vi "set optimum range.vi"(0 "denge degeri":dbl) -> (15 "ok":bool)   [LabVIEW 2014]
uses:
  Sub_VI/show_sensitivity.vi
panel:
  out "cycle":bool
  in  "GPIB In":refnum<visa-resource-name>="GPIB0::8::INSTR"
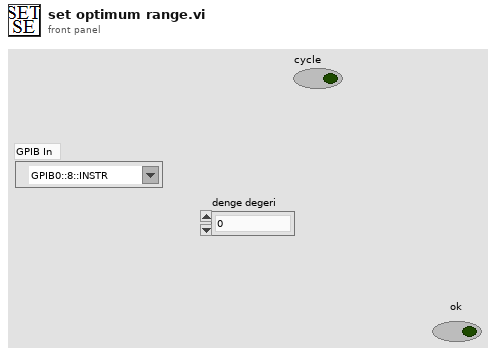
[diagram p1: front panel]
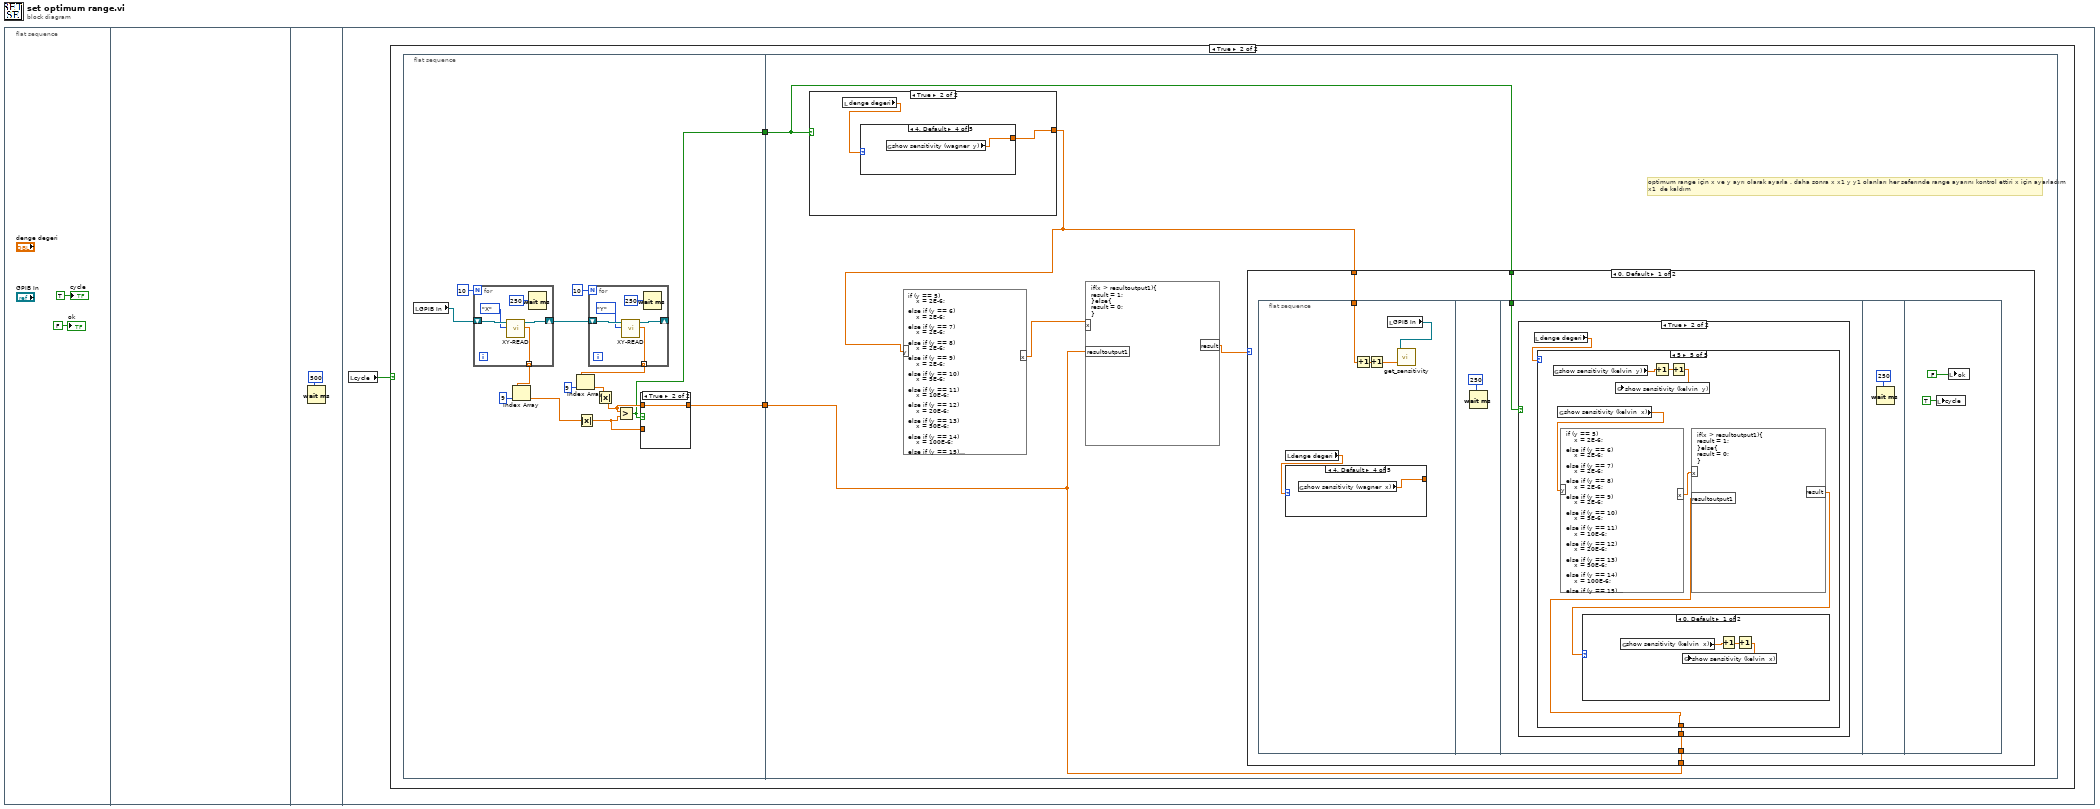
[diagram p0: block diagram]
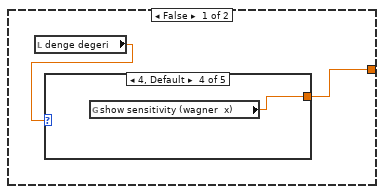
[diagram p4: hidden frame]
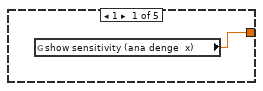
[diagram p5: hidden frame]
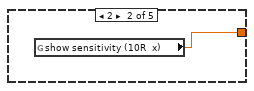
[diagram p6: hidden frame]
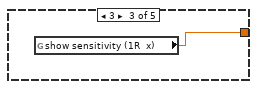
[diagram p7: hidden frame]
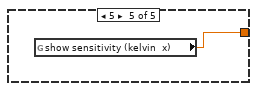
[diagram p8: hidden frame]
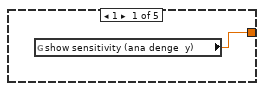
[diagram p9: hidden frame]
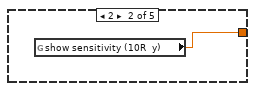
[diagram p10: hidden frame]
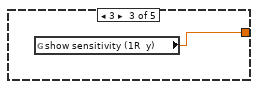
[diagram p11: hidden frame]
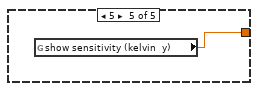
[diagram p12: hidden frame]
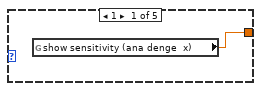
[diagram p13: hidden frame]
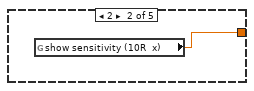
[diagram p14: hidden frame]
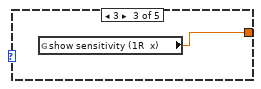
[diagram p15: hidden frame]
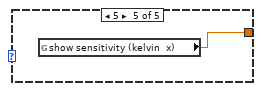
[diagram p16: hidden frame]
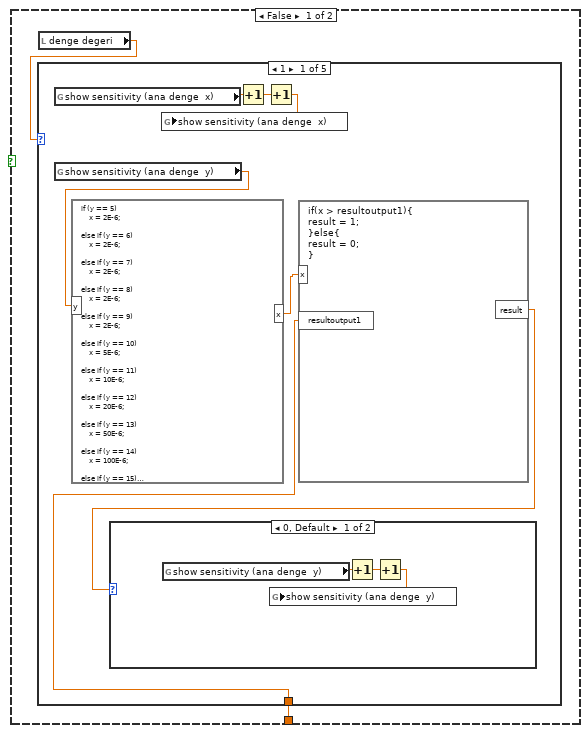
[diagram p17: hidden frame]
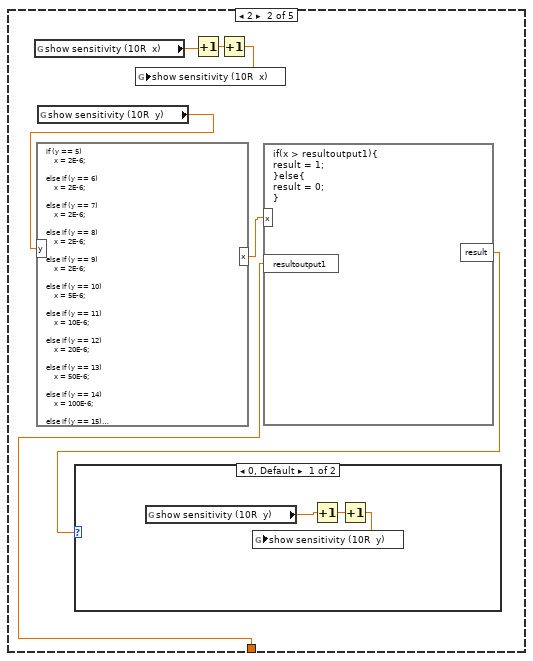
[diagram p19: hidden frame]
diagram:
  n1 = flat-sequence {
    frame #0 {
      "ok" <- FALSE ("Start X")
      "cycle" <- TRUE ("Boolean")
    }
    frame #1 {
    }
    frame #2 {
      n2 = Wait (ms)(milliseconds to wait=u32 500) -> ()  [unwired: 1 out]
    }
    frame #3 {
      n3 = local read "cycle"() -> (w4:bool)
      n4 = case shown="True" w4 {
        frame False {
        }
        frame True {
          n5 = flat-sequence {
            tunnel: [w8] -> w6
            tunnel: [w7] -> w5
            tunnel: w6 -> [w33]
            tunnel: w5 -> [w35]
            frame #0 {
              n6 = local read "GPIB In"() -> (w10:refnum<visa-resource-name>)
              n7 = for {
                N: 10 -> [_]
                shift-right: [w24] -> w9
                shift-left: w10 -> [w25]
                tunnel: [w23] -> w12 mode=indexing
                n8 = call "XY-READ.vi"("X/Y ?"=enum16{"X", "Y"}."X", "SR850 GPIB IN"=w25) -> ("SR850_Reading"=w23:dbl, "SR850 GPIB OUT"=w24:refnum<visa-resource-name>)  [unwired: 7 in, 1 out]
                n9 = Wait (ms)(milliseconds to wait=u32 250) -> ()  [unwired: 1 out]
              }
              n10 = Index Array(array=w12, index=9) -> (element=w20:dbl)
              n11 = Absolute Value(x=w20) -> (abs(x)=w19:dbl)
              n12 = for {
                N: 10 -> [_]
                shift-right: [w31] -> _
                shift-left: w9 -> [w32]
                tunnel: [w30] -> w15 mode=indexing
                n13 = call "XY-READ.vi"("X/Y ?"=enum16{"X", "Y"}."Y", "SR850 GPIB IN"=w32) -> ("SR850_Reading"=w30:dbl, "SR850 GPIB OUT"=w31:refnum<visa-resource-name>)  [unwired: 7 in, 1 out]
                n14 = Wait (ms)(milliseconds to wait=u32 250) -> ()  [unwired: 1 out]
              }
              n15 = Index Array(array=w15, index=9) -> (element=w17:dbl)
              n16 = Absolute Value(x=w17) -> (abs(x)=w18:dbl)
              n17 = Greater?(x=w18, y=w19) -> (0:w7:bool)
              n18 = case shown="True" w7 {
                tunnel: [w26 w27] -> w8
                tunnel: w18 -> [_ w27]
                tunnel: w19 -> [w26 _]
                frame False {
                }
                frame True {
                }
              }
            }
            frame #1 {
              # "optimum range için x ve y ayrı olarak ayarla . daha sonra x x1 y y1 olanları her seferınde range ayarını kontrol ettiri x için ayarladım\nx1  de kaldım"
              n19 = case shown="True" w35 {
                tunnel: [w38 w46] -> w34
                frame False {
                  n20 = local read "denge degeri"() -> (w39:dbl)
                  n21 = case shown="4, Default" w39 {
                    tunnel: [w40 w41 w42 w43 w44] -> w38
                    frame 1 {
                      n22 = global read "show_sensitivity.vi" "show sensitivity (ana denge  x)"() -> (w40:dbl)
                    }
                    frame 2 {
                      n23 = global read "show_sensitivity.vi" "show sensitivity (10R  x)"() -> (w41:dbl)
                    }
                    frame 3 {
                      n24 = global read "show_sensitivity.vi" "show sensitivity (1R  x)"() -> (w42:dbl)
                    }
                    frame 4, Default {
                      n25 = global read "show_sensitivity.vi" "show sensitivity (wagner  x)"() -> (w43:dbl)
                    }
                    frame 5 {
                      n26 = global read "show_sensitivity.vi" "show sensitivity (kelvin  x)"() -> (w44:dbl)
                    }
                  }
                }
                frame True {
                  n27 = local read "denge degeri"() -> (w45:dbl)
                  n28 = case shown="4, Default" w45 {
                    tunnel: [w47 w48 w49 w50 w51] -> w46
                    frame 1 {
                      n29 = global read "show_sensitivity.vi" "show sensitivity (ana denge  y)"() -> (w47:dbl)
                    }
                    frame 2 {
                      n30 = global read "show_sensitivity.vi" "show sensitivity (10R  y)"() -> (w48:dbl)
                    }
                    frame 3 {
                      n31 = global read "show_sensitivity.vi" "show sensitivity (1R  y)"() -> (w49:dbl)
                    }
                    frame 4, Default {
                      n32 = global read "show_sensitivity.vi" "show sensitivity (wagner  y)"() -> (w50:dbl)
                    }
                    frame 5 {
                      n33 = global read "show_sensitivity.vi" "show sensitivity (kelvin  y)"() -> (w51:dbl)
                    }
                  }
                }
              }
              n34 = formula code="if (y == 5) \n    x = 2E-6;\n\nelse if (y == 6) \n    x = 2E-6;\n\nelse if (y == 7) \n    x = 2E-6;\n\nelse if (y == 8) \n    x = 2E-6;\n\nelse if (y == 9) \n    x = 2E-6;\n\nelse if (y == 10) \n    x = 5E-6;\n\nelse if (y == 11) \n    x = 10E-6;\n\nelse if (y == 12) \n    x = 20E-6;\n\nelse if (y == 13) \n    x = 50E-6;\n\nelse if (y == 14) \n    x = 100E-6;\n\nelse if (y == 15) \n    x = 200E-6;\n\nelse if (y == 16) \n    x = 500E-6;\n\nelse if (y == 17) \n    x = 1E-3;\n\nelse if (y == 18) \n    x = 2E-3;\n\nelse if (y == 19) \n    x = 5E-3;\n\nelse if (y == 20) \n    x = 10E-3;\n\nelse if (y == 21) \n    x = 20E-3;\n\nelse if (y == 22) \n    x = 50E-3;\n\nelse if (y == 23) \n    x = 100E-3;\n\nelse if (y == 24) \n    x = 200E-3;\n\nelse if (y == 25) \n    x = 500E-3;\n\nelse if (y == 26) \n    x = 1;\n\nelse \n    x = 1;"("y"=w34) -> ("x"=w36:dbl)
              n35 = formula code="if(x > resultoutput1){\nresult = 1;\n}else{\nresult = 0;\n}"("x"=w36, "resultoutput1"=w33) -> ("result"=w37:dbl)
              n36 = case shown="0, Default" w37 {
                tunnel: w34 -> [w54 _]
                tunnel: w35 -> [w53 _]
                tunnel: w33 -> [w52 _]
                frame 0, Default {
                  n37 = flat-sequence {
                    tunnel: w54 -> [w57]
                    tunnel: w53 -> [w67]
                    tunnel: w52 -> [w66]
                    frame #0 {
                      n38 = local read "denge degeri"() -> (w58:dbl)
                      n39 = case shown="4, Default" w58 {
                        tunnel: [w60 w61 w62 w63 w64] -> _
                        frame 1 {
                          n40 = global read "show_sensitivity.vi" "show sensitivity (ana denge  x)"() -> (w60:dbl)
                        }
                        frame 2 {
                          n41 = global read "show_sensitivity.vi" "show sensitivity (10R  x)"() -> (w61:dbl)
                        }
                        frame 3 {
                          n42 = global read "show_sensitivity.vi" "show sensitivity (1R  x)"() -> (w62:dbl)
                        }
                        frame 4, Default {
                          n43 = global read "show_sensitivity.vi" "show sensitivity (wagner  x)"() -> (w63:dbl)
                        }
                        frame 5 {
                          n44 = global read "show_sensitivity.vi" "show sensitivity (kelvin  x)"() -> (w64:dbl)
                        }
                      }
                      n45 = Increment(x=w57) -> (x+1=w56:dbl)
                      n46 = Increment(x=w56) -> (x+1=w55:dbl)
                      n47 = local read "GPIB In"() -> (w59:refnum<visa-resource-name>)
                      n48 = call "get_sensitivity.vi"("input 1"=w55, "SR850 GPIB In"=w59) -> ()  [unwired: 8 in, 2 out]
                    }
                    frame #1 {
                      n49 = Wait (ms)(milliseconds to wait=u32 250) -> ()  [unwired: 1 out]
                    }
                    frame #2 {
                      n50 = case shown="True" w67 {
                        tunnel: w66 -> [w68 w120]
                        frame False {
                          n51 = local read "denge degeri"() -> (w69:dbl)
                          n52 = case shown="1" w69 {
                            tunnel: w68 -> [w70 w80 w90 w100 w110]
                            frame 1 {
                              n53 = global read "show_sensitivity.vi" "show sensitivity (ana denge  x)"() -> (w76:dbl)
                              n54 = global read "show_sensitivity.vi" "show sensitivity (ana denge  y)"() -> (w73:dbl)
                              n55 = formula code="if (y == 5) \n    x = 2E-6;\n\nelse if (y == 6) \n    x = 2E-6;\n\nelse if (y == 7) \n    x = 2E-6;\n\nelse if (y == 8) \n    x = 2E-6;\n\nelse if (y == 9) \n    x = 2E-6;\n\nelse if (y == 10) \n    x = 5E-6;\n\nelse if (y == 11) \n    x = 10E-6;\n\nelse if (y == 12) \n    x = 20E-6;\n\nelse if (y == 13) \n    x = 50E-6;\n\nelse if (y == 14) \n    x = 100E-6;\n\nelse if (y == 15) \n    x = 200E-6;\n\nelse if (y == 16) \n    x = 500E-6;\n\nelse if (y == 17) \n    x = 1E-3;\n\nelse if (y == 18) \n    x = 2E-3;\n\nelse if (y == 19) \n    x = 5E-3;\n\nelse if (y == 20) \n    x = 10E-3;\n\nelse if (y == 21) \n    x = 20E-3;\n\nelse if (y == 22) \n    x = 50E-3;\n\nelse if (y == 23) \n    x = 100E-3;\n\nelse if (y == 24) \n    x = 200E-3;\n\nelse if (y == 25) \n    x = 500E-3;\n\nelse if (y == 26) \n    x = 1;\n\nelse \n    x = 1;"("y"=w73) -> ("x"=w72:dbl)
                              n56 = Increment(x=w76) -> (x+1=w75:dbl)
                              n57 = Increment(x=w75) -> (x+1=w74:dbl)
                              n58 = global write "show_sensitivity.vi" "show sensitivity (ana denge  x)"(w74) -> ()
                              n59 = formula code="if(x > resultoutput1){\nresult = 1;\n}else{\nresult = 0;\n}"("x"=w72, "resultoutput1"=w70) -> ("result"=w71:dbl)
                              n60 = case shown="0, Default" w71 {
                                frame 0, Default {
                                n61 = global read "show_sensitivity.vi" "show sensitivity (ana denge  y)"() -> (w77:dbl)
                                n62 = Increment(x=w77) -> (x+1=w78:dbl)
                                n63 = Increment(x=w78) -> (x+1=w79:dbl)
                                n64 = global write "show_sensitivity.vi" "show sensitivity (ana denge  y)"(w79) -> ()
                                }
                                frame 1 {
                                }
                              }
                            }
                            frame 2 {
                              n65 = global read "show_sensitivity.vi" "show sensitivity (10R  x)"() -> (w86:dbl)
                              n66 = global read "show_sensitivity.vi" "show sensitivity (10R  y)"() -> (w83:dbl)
                              n67 = formula code="if (y == 5) \n    x = 2E-6;\n\nelse if (y == 6) \n    x = 2E-6;\n\nelse if (y == 7) \n    x = 2E-6;\n\nelse if (y == 8) \n    x = 2E-6;\n\nelse if (y == 9) \n    x = 2E-6;\n\nelse if (y == 10) \n    x = 5E-6;\n\nelse if (y == 11) \n    x = 10E-6;\n\nelse if (y == 12) \n    x = 20E-6;\n\nelse if (y == 13) \n    x = 50E-6;\n\nelse if (y == 14) \n    x = 100E-6;\n\nelse if (y == 15) \n    x = 200E-6;\n\nelse if (y == 16) \n    x = 500E-6;\n\nelse if (y == 17) \n    x = 1E-3;\n\nelse if (y == 18) \n    x = 2E-3;\n\nelse if (y == 19) \n    x = 5E-3;\n\nelse if (y == 20) \n    x = 10E-3;\n\nelse if (y == 21) \n    x = 20E-3;\n\nelse if (y == 22) \n    x = 50E-3;\n\nelse if (y == 23) \n    x = 100E-3;\n\nelse if (y == 24) \n    x = 200E-3;\n\nelse if (y == 25) \n    x = 500E-3;\n\nelse if (y == 26) \n    x = 1;\n\nelse \n    x = 1;"("y"=w83) -> ("x"=w82:dbl)
                              n68 = Increment(x=w86) -> (x+1=w85:dbl)
                              n69 = Increment(x=w85) -> (x+1=w84:dbl)
                              n70 = global write "show_sensitivity.vi" "show sensitivity (10R  x)"(w84) -> ()
                              n71 = formula code="if(x > resultoutput1){\nresult = 1;\n}else{\nresult = 0;\n}"("x"=w82, "resultoutput1"=w80) -> ("result"=w81:dbl)
                              n72 = case shown="0, Default" w81 {
                                frame 0, Default {
                                n73 = global read "show_sensitivity.vi" "show sensitivity (10R  y)"() -> (w87:dbl)
                                n74 = Increment(x=w87) -> (x+1=w88:dbl)
                                n75 = Increment(x=w88) -> (x+1=w89:dbl)
                                n76 = global write "show_sensitivity.vi" "show sensitivity (10R  y)"(w89) -> ()
                                }
                                frame 1 {
                                }
                              }
                            }
                            frame 3 {
                              n77 = global read "show_sensitivity.vi" "show sensitivity (1R  y)"() -> (w93:dbl)
                              n78 = formula code="if (y == 5) \n    x = 2E-6;\n\nelse if (y == 6) \n    x = 2E-6;\n\nelse if (y == 7) \n    x = 2E-6;\n\nelse if (y == 8) \n    x = 2E-6;\n\nelse if (y == 9) \n    x = 2E-6;\n\nelse if (y == 10) \n    x = 5E-6;\n\nelse if (y == 11) \n    x = 10E-6;\n\nelse if (y == 12) \n    x = 20E-6;\n\nelse if (y == 13) \n    x = 50E-6;\n\nelse if (y == 14) \n    x = 100E-6;\n\nelse if (y == 15) \n    x = 200E-6;\n\nelse if (y == 16) \n    x = 500E-6;\n\nelse if (y == 17) \n    x = 1E-3;\n\nelse if (y == 18) \n    x = 2E-3;\n\nelse if (y == 19) \n    x = 5E-3;\n\nelse if (y == 20) \n    x = 10E-3;\n\nelse if (y == 21) \n    x = 20E-3;\n\nelse if (y == 22) \n    x = 50E-3;\n\nelse if (y == 23) \n    x = 100E-3;\n\nelse if (y == 24) \n    x = 200E-3;\n\nelse if (y == 25) \n    x = 500E-3;\n\nelse if (y == 26) \n    x = 1;\n\nelse \n    x = 1;"("y"=w93) -> ("x"=w92:dbl)
                              n79 = global read "show_sensitivity.vi" "show sensitivity (1R  x)"() -> (w96:dbl)
                              n80 = Increment(x=w96) -> (x+1=w95:dbl)
                              n81 = Increment(x=w95) -> (x+1=w94:dbl)
                              n82 = global write "show_sensitivity.vi" "show sensitivity (1R  x)"(w94) -> ()
                              n83 = formula code="if(x > resultoutput1){\nresult = 1;\n}else{\nresult = 0;\n}"("x"=w92, "resultoutput1"=w90) -> ("result"=w91:dbl)
                              n84 = case shown="0, Default" w91 {
                                frame 0, Default {
                                n85 = global read "show_sensitivity.vi" "show sensitivity (1R  y)"() -> (w97:dbl)
                                n86 = Increment(x=w97) -> (x+1=w98:dbl)
                                n87 = Increment(x=w98) -> (x+1=w99:dbl)
                                n88 = global write "show_sensitivity.vi" "show sensitivity (1R  y)"(w99) -> ()
                                }
                                frame 1 {
                                }
                              }
                            }
                            frame 4, Default {
                              n89 = global read "show_sensitivity.vi" "show sensitivity (wagner  x)"() -> (w106:dbl)
                              n90 = global read "show_sensitivity.vi" "show sensitivity (wagner  y)"() -> (w103:dbl)
                              n91 = formula code="if (y == 5) \n    x = 2E-6;\n\nelse if (y == 6) \n    x = 2E-6;\n\nelse if (y == 7) \n    x = 2E-6;\n\nelse if (y == 8) \n    x = 2E-6;\n\nelse if (y == 9) \n    x = 2E-6;\n\nelse if (y == 10) \n    x = 5E-6;\n\nelse if (y == 11) \n    x = 10E-6;\n\nelse if (y == 12) \n    x = 20E-6;\n\nelse if (y == 13) \n    x = 50E-6;\n\nelse if (y == 14) \n    x = 100E-6;\n\nelse if (y == 15) \n    x = 200E-6;\n\nelse if (y == 16) \n    x = 500E-6;\n\nelse if (y == 17) \n    x = 1E-3;\n\nelse if (y == 18) \n    x = 2E-3;\n\nelse if (y == 19) \n    x = 5E-3;\n\nelse if (y == 20) \n    x = 10E-3;\n\nelse if (y == 21) \n    x = 20E-3;\n\nelse if (y == 22) \n    x = 50E-3;\n\nelse if (y == 23) \n    x = 100E-3;\n\nelse if (y == 24) \n    x = 200E-3;\n\nelse if (y == 25) \n    x = 500E-3;\n\nelse if (y == 26) \n    x = 1;\n\nelse \n    x = 1;"("y"=w103) -> ("x"=w102:dbl)
                              n92 = Increment(x=w106) -> (x+1=w105:dbl)
                              n93 = Increment(x=w105) -> (x+1=w104:dbl)
                              n94 = global write "show_sensitivity.vi" "show sensitivity (wagner  x)"(w104) -> ()
                              n95 = formula code="if(x > resultoutput1){\nresult = 1;\n}else{\nresult = 0;\n}"("x"=w102, "resultoutput1"=w100) -> ("result"=w101:dbl)
                              n96 = case shown="0, Default" w101 {
                                frame 0, Default {
                                n97 = global read "show_sensitivity.vi" "show sensitivity (wagner  y)"() -> (w107:dbl)
                                n98 = Increment(x=w107) -> (x+1=w108:dbl)
                                n99 = Increment(x=w108) -> (x+1=w109:dbl)
                                n100 = global write "show_sensitivity.vi" "show sensitivity (wagner  y)"(w109) -> ()
                                }
                                frame 1 {
                                }
                              }
                            }
                            frame 5 {
                              n101 = global read "show_sensitivity.vi" "show sensitivity (kelvin  x)"() -> (w116:dbl)
                              n102 = global read "show_sensitivity.vi" "show sensitivity (kelvin  y)"() -> (w113:dbl)
                              n103 = formula code="if (y == 5) \n    x = 2E-6;\n\nelse if (y == 6) \n    x = 2E-6;\n\nelse if (y == 7) \n    x = 2E-6;\n\nelse if (y == 8) \n    x = 2E-6;\n\nelse if (y == 9) \n    x = 2E-6;\n\nelse if (y == 10) \n    x = 5E-6;\n\nelse if (y == 11) \n    x = 10E-6;\n\nelse if (y == 12) \n    x = 20E-6;\n\nelse if (y == 13) \n    x = 50E-6;\n\nelse if (y == 14) \n    x = 100E-6;\n\nelse if (y == 15) \n    x = 200E-6;\n\nelse if (y == 16) \n    x = 500E-6;\n\nelse if (y == 17) \n    x = 1E-3;\n\nelse if (y == 18) \n    x = 2E-3;\n\nelse if (y == 19) \n    x = 5E-3;\n\nelse if (y == 20) \n    x = 10E-3;\n\nelse if (y == 21) \n    x = 20E-3;\n\nelse if (y == 22) \n    x = 50E-3;\n\nelse if (y == 23) \n    x = 100E-3;\n\nelse if (y == 24) \n    x = 200E-3;\n\nelse if (y == 25) \n    x = 500E-3;\n\nelse if (y == 26) \n    x = 1;\n\nelse \n    x = 1;"("y"=w113) -> ("x"=w112:dbl)
                              n104 = Increment(x=w116) -> (x+1=w115:dbl)
                              n105 = Increment(x=w115) -> (x+1=w114:dbl)
                              n106 = global write "show_sensitivity.vi" "show sensitivity (kelvin  x)"(w114) -> ()
                              n107 = formula code="if(x > resultoutput1){\nresult = 1;\n}else{\nresult = 0;\n}"("x"=w112, "resultoutput1"=w110) -> ("result"=w111:dbl)
                              n108 = case shown="0, Default" w111 {
                                frame 0, Default {
                                n109 = global read "show_sensitivity.vi" "show sensitivity (kelvin  y)"() -> (w117:dbl)
                                n110 = Increment(x=w117) -> (x+1=w118:dbl)
                                n111 = Increment(x=w118) -> (x+1=w119:dbl)
                                n112 = global write "show_sensitivity.vi" "show sensitivity (kelvin  y)"(w119) -> ()
                                }
                                frame 1 {
                                }
                              }
                            }
                          }
                        }
                        frame True {
                          n113 = local read "denge degeri"() -> (w121:dbl)
                          n114 = case shown="5" w121 {
                            tunnel: w120 -> [w122 w132 w142 w152 w162]
                            frame 1 {
                              n115 = global read "show_sensitivity.vi" "show sensitivity (ana denge  y)"() -> (w126:dbl)
                              n116 = global read "show_sensitivity.vi" "show sensitivity (ana denge  x)"() -> (w125:dbl)
                              n117 = formula code="if (y == 5) \n    x = 2E-6;\n\nelse if (y == 6) \n    x = 2E-6;\n\nelse if (y == 7) \n    x = 2E-6;\n\nelse if (y == 8) \n    x = 2E-6;\n\nelse if (y == 9) \n    x = 2E-6;\n\nelse if (y == 10) \n    x = 5E-6;\n\nelse if (y == 11) \n    x = 10E-6;\n\nelse if (y == 12) \n    x = 20E-6;\n\nelse if (y == 13) \n    x = 50E-6;\n\nelse if (y == 14) \n    x = 100E-6;\n\nelse if (y == 15) \n    x = 200E-6;\n\nelse if (y == 16) \n    x = 500E-6;\n\nelse if (y == 17) \n    x = 1E-3;\n\nelse if (y == 18) \n    x = 2E-3;\n\nelse if (y == 19) \n    x = 5E-3;\n\nelse if (y == 20) \n    x = 10E-3;\n\nelse if (y == 21) \n    x = 20E-3;\n\nelse if (y == 22) \n    x = 50E-3;\n\nelse if (y == 23) \n    x = 100E-3;\n\nelse if (y == 24) \n    x = 200E-3;\n\nelse if (y == 25) \n    x = 500E-3;\n\nelse if (y == 26) \n    x = 1;\n\nelse \n    x = 1;"("y"=w125) -> ("x"=w124:dbl)
                              n118 = Increment(x=w126) -> (x+1=w127:dbl)
                              n119 = Increment(x=w127) -> (x+1=w128:dbl)
                              n120 = global write "show_sensitivity.vi" "show sensitivity (ana denge  y)"(w128) -> ()
                              n121 = formula code="if(x > resultoutput1){\nresult = 1;\n}else{\nresult = 0;\n}"("x"=w124, "resultoutput1"=w122) -> ("result"=w123:dbl)
                              n122 = case shown="0, Default" w123 {
                                frame 0, Default {
                                n123 = global read "show_sensitivity.vi" "show sensitivity (ana denge  x)"() -> (w129:dbl)
                                n124 = Increment(x=w129) -> (x+1=w130:dbl)
                                n125 = Increment(x=w130) -> (x+1=w131:dbl)
                                n126 = global write "show_sensitivity.vi" "show sensitivity (ana denge  x)"(w131) -> ()
                                }
                                frame 1 {
                                }
                              }
                            }
                            frame 2 {
                              n127 = global read "show_sensitivity.vi" "show sensitivity (10R  y)"() -> (w136:dbl)
                              n128 = global read "show_sensitivity.vi" "show sensitivity (10R  x)"() -> (w135:dbl)
                              n129 = formula code="if (y == 5) \n    x = 2E-6;\n\nelse if (y == 6) \n    x = 2E-6;\n\nelse if (y == 7) \n    x = 2E-6;\n\nelse if (y == 8) \n    x = 2E-6;\n\nelse if (y == 9) \n    x = 2E-6;\n\nelse if (y == 10) \n    x = 5E-6;\n\nelse if (y == 11) \n    x = 10E-6;\n\nelse if (y == 12) \n    x = 20E-6;\n\nelse if (y == 13) \n    x = 50E-6;\n\nelse if (y == 14) \n    x = 100E-6;\n\nelse if (y == 15) \n    x = 200E-6;\n\nelse if (y == 16) \n    x = 500E-6;\n\nelse if (y == 17) \n    x = 1E-3;\n\nelse if (y == 18) \n    x = 2E-3;\n\nelse if (y == 19) \n    x = 5E-3;\n\nelse if (y == 20) \n    x = 10E-3;\n\nelse if (y == 21) \n    x = 20E-3;\n\nelse if (y == 22) \n    x = 50E-3;\n\nelse if (y == 23) \n    x = 100E-3;\n\nelse if (y == 24) \n    x = 200E-3;\n\nelse if (y == 25) \n    x = 500E-3;\n\nelse if (y == 26) \n    x = 1;\n\nelse \n    x = 1;"("y"=w135) -> ("x"=w134:dbl)
                              n130 = Increment(x=w136) -> (x+1=w137:dbl)
                              n131 = Increment(x=w137) -> (x+1=w138:dbl)
                              n132 = global write "show_sensitivity.vi" "show sensitivity (10R  y)"(w138) -> ()
                              n133 = formula code="if(x > resultoutput1){\nresult = 1;\n}else{\nresult = 0;\n}"("x"=w134, "resultoutput1"=w132) -> ("result"=w133:dbl)
                              n134 = case shown="0, Default" w133 {
                                frame 0, Default {
                                n135 = global read "show_sensitivity.vi" "show sensitivity (10R  x)"() -> (w139:dbl)
                                n136 = Increment(x=w139) -> (x+1=w140:dbl)
                                n137 = Increment(x=w140) -> (x+1=w141:dbl)
                                n138 = global write "show_sensitivity.vi" "show sensitivity (10R  x)"(w141) -> ()
                                }
                                frame 1 {
                                }
                              }
                            }
                            frame 3 {
                              n139 = global read "show_sensitivity.vi" "show sensitivity (1R  y)"() -> (w146:dbl)
                              n140 = global read "show_sensitivity.vi" "show sensitivity (1R  x)"() -> (w145:dbl)
                              n141 = formula code="if (y == 5) \n    x = 2E-6;\n\nelse if (y == 6) \n    x = 2E-6;\n\nelse if (y == 7) \n    x = 2E-6;\n\nelse if (y == 8) \n    x = 2E-6;\n\nelse if (y == 9) \n    x = 2E-6;\n\nelse if (y == 10) \n    x = 5E-6;\n\nelse if (y == 11) \n    x = 10E-6;\n\nelse if (y == 12) \n    x = 20E-6;\n\nelse if (y == 13) \n    x = 50E-6;\n\nelse if (y == 14) \n    x = 100E-6;\n\nelse if (y == 15) \n    x = 200E-6;\n\nelse if (y == 16) \n    x = 500E-6;\n\nelse if (y == 17) \n    x = 1E-3;\n\nelse if (y == 18) \n    x = 2E-3;\n\nelse if (y == 19) \n    x = 5E-3;\n\nelse if (y == 20) \n    x = 10E-3;\n\nelse if (y == 21) \n    x = 20E-3;\n\nelse if (y == 22) \n    x = 50E-3;\n\nelse if (y == 23) \n    x = 100E-3;\n\nelse if (y == 24) \n    x = 200E-3;\n\nelse if (y == 25) \n    x = 500E-3;\n\nelse if (y == 26) \n    x = 1;\n\nelse \n    x = 1;"("y"=w145) -> ("x"=w144:dbl)
                              n142 = Increment(x=w146) -> (x+1=w147:dbl)
                              n143 = Increment(x=w147) -> (x+1=w148:dbl)
                              n144 = global write "show_sensitivity.vi" "show sensitivity (1R  y)"(w148) -> ()
                              n145 = formula code="if(x > resultoutput1){\nresult = 1;\n}else{\nresult = 0;\n}"("x"=w144, "resultoutput1"=w142) -> ("result"=w143:dbl)
                              n146 = case shown="0, Default" w143 {
                                frame 0, Default {
                                n147 = global read "show_sensitivity.vi" "show sensitivity (1R  x)"() -> (w149:dbl)
                                n148 = Increment(x=w149) -> (x+1=w150:dbl)
                                n149 = Increment(x=w150) -> (x+1=w151:dbl)
                                n150 = global write "show_sensitivity.vi" "show sensitivity (1R  x)"(w151) -> ()
                                }
                                frame 1 {
                                }
                              }
                            }
                            frame 4, Default {
                              n151 = global read "show_sensitivity.vi" "show sensitivity (wagner  y)"() -> (w156:dbl)
                              n152 = global read "show_sensitivity.vi" "show sensitivity (wagner  x)"() -> (w155:dbl)
                              n153 = formula code="if (y == 5) \n    x = 2E-6;\n\nelse if (y == 6) \n    x = 2E-6;\n\nelse if (y == 7) \n    x = 2E-6;\n\nelse if (y == 8) \n    x = 2E-6;\n\nelse if (y == 9) \n    x = 2E-6;\n\nelse if (y == 10) \n    x = 5E-6;\n\nelse if (y == 11) \n    x = 10E-6;\n\nelse if (y == 12) \n    x = 20E-6;\n\nelse if (y == 13) \n    x = 50E-6;\n\nelse if (y == 14) \n    x = 100E-6;\n\nelse if (y == 15) \n    x = 200E-6;\n\nelse if (y == 16) \n    x = 500E-6;\n\nelse if (y == 17) \n    x = 1E-3;\n\nelse if (y == 18) \n    x = 2E-3;\n\nelse if (y == 19) \n    x = 5E-3;\n\nelse if (y == 20) \n    x = 10E-3;\n\nelse if (y == 21) \n    x = 20E-3;\n\nelse if (y == 22) \n    x = 50E-3;\n\nelse if (y == 23) \n    x = 100E-3;\n\nelse if (y == 24) \n    x = 200E-3;\n\nelse if (y == 25) \n    x = 500E-3;\n\nelse if (y == 26) \n    x = 1;\n\nelse \n    x = 1;"("y"=w155) -> ("x"=w154:dbl)
                              n154 = Increment(x=w156) -> (x+1=w157:dbl)
                              n155 = Increment(x=w157) -> (x+1=w158:dbl)
                              n156 = global write "show_sensitivity.vi" "show sensitivity (wagner  y)"(w158) -> ()
                              n157 = formula code="if(x > resultoutput1){\nresult = 1;\n}else{\nresult = 0;\n}"("x"=w154, "resultoutput1"=w152) -> ("result"=w153:dbl)
                              n158 = case shown="0, Default" w153 {
                                frame 0, Default {
                                n159 = global read "show_sensitivity.vi" "show sensitivity (wagner  x)"() -> (w159:dbl)
                                n160 = Increment(x=w159) -> (x+1=w160:dbl)
                                n161 = Increment(x=w160) -> (x+1=w161:dbl)
                                n162 = global write "show_sensitivity.vi" "show sensitivity (wagner  x)"(w161) -> ()
                                }
                                frame 1 {
                                }
                              }
                            }
                            frame 5 {
                              n163 = global read "show_sensitivity.vi" "show sensitivity (kelvin  y)"() -> (w166:dbl)
                              n164 = global read "show_sensitivity.vi" "show sensitivity (kelvin  x)"() -> (w165:dbl)
                              n165 = formula code="if (y == 5) \n    x = 2E-6;\n\nelse if (y == 6) \n    x = 2E-6;\n\nelse if (y == 7) \n    x = 2E-6;\n\nelse if (y == 8) \n    x = 2E-6;\n\nelse if (y == 9) \n    x = 2E-6;\n\nelse if (y == 10) \n    x = 5E-6;\n\nelse if (y == 11) \n    x = 10E-6;\n\nelse if (y == 12) \n    x = 20E-6;\n\nelse if (y == 13) \n    x = 50E-6;\n\nelse if (y == 14) \n    x = 100E-6;\n\nelse if (y == 15) \n    x = 200E-6;\n\nelse if (y == 16) \n    x = 500E-6;\n\nelse if (y == 17) \n    x = 1E-3;\n\nelse if (y == 18) \n    x = 2E-3;\n\nelse if (y == 19) \n    x = 5E-3;\n\nelse if (y == 20) \n    x = 10E-3;\n\nelse if (y == 21) \n    x = 20E-3;\n\nelse if (y == 22) \n    x = 50E-3;\n\nelse if (y == 23) \n    x = 100E-3;\n\nelse if (y == 24) \n    x = 200E-3;\n\nelse if (y == 25) \n    x = 500E-3;\n\nelse if (y == 26) \n    x = 1;\n\nelse \n    x = 1;"("y"=w165) -> ("x"=w164:dbl)
                              n166 = Increment(x=w166) -> (x+1=w167:dbl)
                              n167 = Increment(x=w167) -> (x+1=w168:dbl)
                              n168 = global write "show_sensitivity.vi" "show sensitivity (kelvin  y)"(w168) -> ()
                              n169 = formula code="if(x > resultoutput1){\nresult = 1;\n}else{\nresult = 0;\n}"("x"=w164, "resultoutput1"=w162) -> ("result"=w163:dbl)
                              n170 = case shown="0, Default" w163 {
                                frame 0, Default {
                                n171 = global read "show_sensitivity.vi" "show sensitivity (kelvin  x)"() -> (w169:dbl)
                                n172 = Increment(x=w169) -> (x+1=w170:dbl)
                                n173 = Increment(x=w170) -> (x+1=w171:dbl)
                                n174 = global write "show_sensitivity.vi" "show sensitivity (kelvin  x)"(w171) -> ()
                                }
                                frame 1 {
                                }
                              }
                            }
                          }
                        }
                      }
                    }
                    frame #3 {
                      n175 = Wait (ms)(milliseconds to wait=u32 250) -> ()  [unwired: 1 out]
                    }
                    frame #4 {
                      n176 = local write "cycle"(TRUE ("cycle")) -> ()
                      n177 = local write "ok"(FALSE ("Start X")) -> ()
                    }
                  }
                }
                frame 1 {
                  n178 = local write "cycle"(FALSE ("Start X")) -> ()
                  n179 = local write "ok"(TRUE ("Start X")) -> ()
                }
              }
            }
          }
        }
      }
    }
  }
